vi "Vision Processing.vi"() -> ()   [LabVIEW 2011]
doc: "This VI runs in parallel to other tasks. It gets images from the camera, processes them for color or shape and use that information to affect robot behavior."
panel:
  out "Particle Measurements (Pixels) (Particle Analysis 1)":dbl[][](array[numeric]) format="%.2f"
  out "Number of Particles (Particle Analysis 1)":i32
  out "Numeric":i32
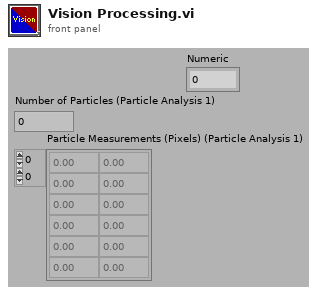
[diagram p1: front panel]
types:
  T1 = typedef "Image Type" = u32
  T2 = typedef "WPI_CameraDevRef.ctl" = cluster{"Camera Address":string, "CameraStatus":errorcluster, "Acquire Image Notifier":refnum<notifier>}
  T3 = typedef "IMAQ Image.ctl" = refnum<image>
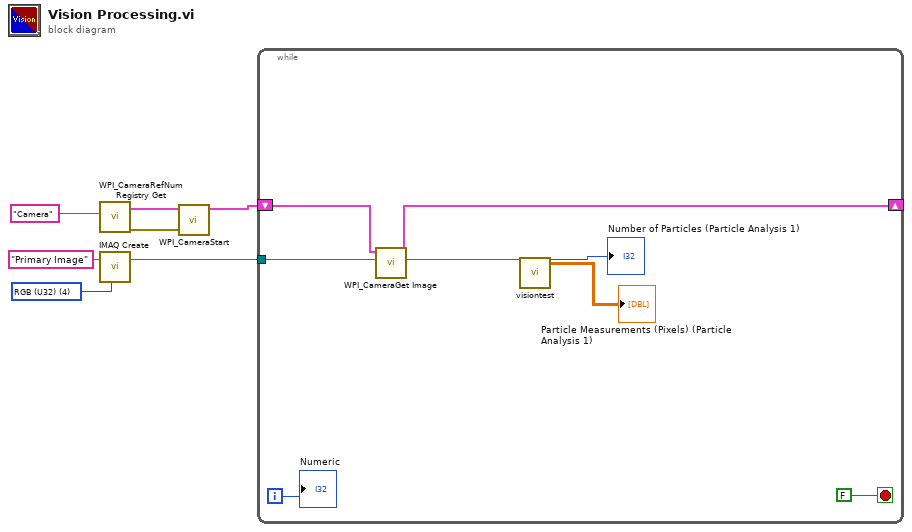
[diagram p0: block diagram]
diagram:
  w7 = T1 4 items=["Grayscale (U8)", "Grayscale (I16)", "Grayscale (SGL)", "Complex (CSG)", "RGB (U32)", "HSL (U32)", "RGB (U64)"] ("Image Type")
  n1 = call <vilib>:"WPI_CameraRefNum Registry Get.vi"("refnum name"="Camera") -> ("error out"=w2:errorcluster, "CameraDevRef"=w3:T2)  [unwired: 1 in, 8 out]
  n2 = call "IMAQ Create"("Image Name"="Primary Image", "Image Type"=w7) -> ("New Image"=w5:T3)  [unwired: 2 in, 2 out]
  n3 = call <vilib>:"WPI_CameraStart.vi"("error in (no error)"=w2, "CameraDevRef"=w3) -> ("CameraDevRef Out"=w1:T2)  [unwired: 9 out]
  n4 = while {
    shift-right: [w14] -> _
    shift-left: w1 -> [w12]
    tunnel: w5 -> [w13]
    i -> [w11]
    stop <- FALSE stop-if-true
    n5 = call <vilib>:"WPI_CameraGet Image.vi"("Image"=w13, "CameraDevRef"=w12) -> ("Image Out"=w10:T3, "CameraDevRef Out"=w14:T2)  [unwired: 1 in, 7 out]
    n6 = call "visiontest.vi"("Image Src"=w10) -> ("Number of Particles (Particle Analysis 1)"=→"Number of Particles (Particle Analysis 1)":i32, "Particle Measurements (Pixels) (Particle Analysis 1)"=→"Particle Measurements (Pixels) (Particle Analysis 1)":dbl[][])  [unwired: 1 in, 24 out]
    "Numeric" <- w11
  }
